vi "Signal Extension.vi"(9 "extension length":i32, 10 "X extension type":u16(ring) items=["Zero padding", "Symmetric", "Periodic"], 11 "X In":dbl[](array[numeric])) -> (0 "error":i32, 1 "Final Condition":dbl[](array[numeric]), 2 "X Out":dbl[](array[numeric]), 3 "Initial Condition":dbl[](array[numeric]))   [LabVIEW 2017, in "NI_AAL_Filter.lvlib"]
uses:
  <vilib>/Analysis/NI_AAL_Filter.lvlib
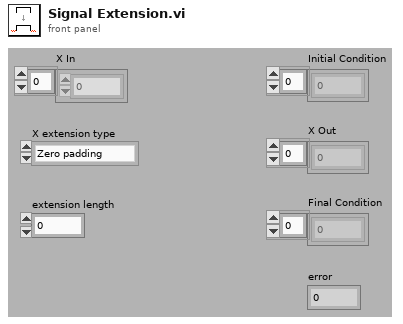
[diagram p1: front panel]
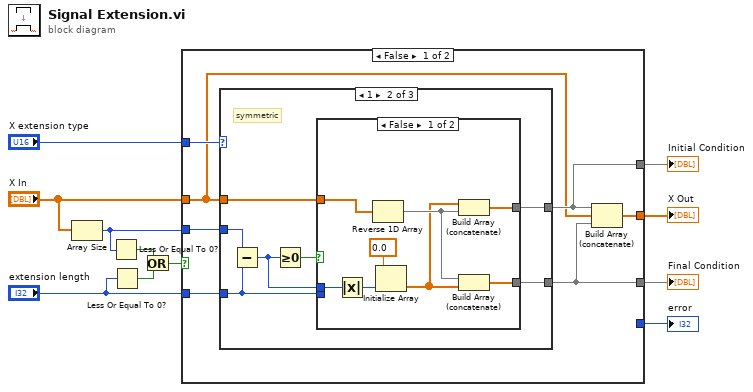
[diagram p0: block diagram]
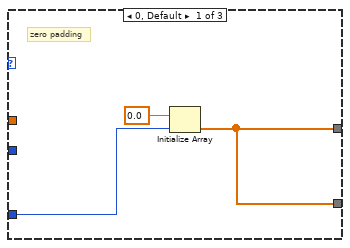
[diagram p2: hidden frame]
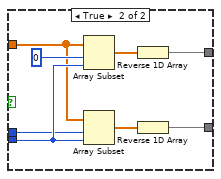
[diagram p3: hidden frame]
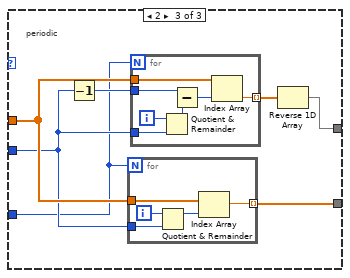
[diagram p4: hidden frame]
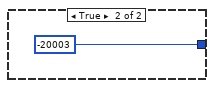
[diagram p5: hidden frame]
diagram:
  n1 = Array Size(array="X In") -> (size(s)=w6:i32)
  n2 = Less Or Equal To 0?(x=w6) -> (x <= 0?=w3:bool)
  n3 = Less Or Equal To 0?(x="extension length") -> (x <= 0?=w2:bool)
  n4 = Or(x=w3, y=w2) -> (x .or. y?=w4:bool)
  n5 = case shown="False" w4 {
    tunnel: "X extension type" -> [w18 _]
    tunnel: [w17 _] -> w10
    tunnel: [w16 _] -> w9
    tunnel: [w15 _] -> w8
    tunnel: "X In" -> [w12 _]
    tunnel: w6 -> [w14 _]
    tunnel: "extension length" -> [w13 _]
    tunnel: [_ -20003] -> w1
    frame False {
      n6 = case shown="1" w18 {
        tunnel: w12 -> [_ w25 w50]
        tunnel: [w20 w26 w51] -> w17
        tunnel: [w20 w27 w46] -> w15
        tunnel: w14 -> [_ w24 w49]
        tunnel: w13 -> [w19 w22 w45]
        frame 0, Default {
          # "zero padding"
          n7 = Initialize Array(0.0, w19) -> (w20:dbl[])
        }
        frame 1 {
          # "symmetric"
          n8 = Subtract(x=w24, y=w22) -> (x-y=w23:i32)
          n9 = Greater Or Equal To 0?(x=w23) -> (x >= 0?=w28:bool)
          n10 = case shown="False" w28 {
            tunnel: [w33 w38] -> w27
            tunnel: [w31 w37] -> w26
            tunnel: w22 -> [_ w41]
            tunnel: w25 -> [w29 w40]
            tunnel: w23 -> [w36 w39]
            frame False {
              n11 = Absolute Value(x=w36) -> (abs(x)=w35:i32)
              n12 = Reverse 1D Array(array=w29) -> (reversed array=w32:dbl[])
              n13 = Initialize Array(0.0 ("element"), w35) -> (w30:dbl[])
              n14 = Build Array (concatenate)(w30, w32) -> (w33:dbl[])
              n15 = Build Array (concatenate)(w32, w30) -> (w31:dbl[])
            }
            frame True {
              n16 = Array Subset(array=w40, index=0, length=w41) -> (w43:dbl[])
              n17 = Array Subset(array=w40, index=w39, length=w41) -> (w44:dbl[])
              n18 = Reverse 1D Array(array=w43) -> (reversed array=w38:dbl[])
              n19 = Reverse 1D Array(array=w44) -> (reversed array=w37:dbl[])
            }
          }
        }
        frame 2 {
          # "periodic"
          n20 = Decrement(x=w49) -> (x-1=w48:i32)
          n21 = for {
            N: w45 -> [_]
            tunnel: w50 -> [w63]
            tunnel: [w62] -> w51 mode=indexing
            tunnel: w49 -> [w60]
            i -> [w61]
            n22 = Quotient & Remainder(x=w61, y=w60) -> (x-y*floor(x/y)=w59:i32)  [unwired: 1 out]
            n23 = Index Array(array=w63, index=w59) -> (element=w62:dbl)
          }
          n24 = for {
            N: w45 -> [_]
            tunnel: w50 -> [w58]
            tunnel: [w57] -> w47 mode=indexing
            tunnel: w49 -> [w56]
            tunnel: w48 -> [w53]
            i -> [w55]
            n25 = Quotient & Remainder(x=w55, y=w56) -> (x-y*floor(x/y)=w54:i32)  [unwired: 1 out]
            n26 = Subtract(x=w53, y=w54) -> (x-y=w52:i32)
            n27 = Index Array(array=w58, index=w52) -> (element=w57:dbl)
          }
          n28 = Reverse 1D Array(array=w47) -> (reversed array=w46:dbl[])
        }
      }
      n29 = Build Array (concatenate)(w15, w12, w17) -> (w16:dbl[])
    }
    frame True {
    }
  }
  "Final Condition" <- w10
  "Initial Condition" <- w8
  "X Out" <- w9
  "error" <- w1
